vi "Stitch DAQ and Scope Data.vi"(8 "error in (no error)":errorcluster, 10 "Scope Ch1 (final A-B)":dbl[][](array[numeric]), 11 "DAQ DOD (final)":dbl[][](array[numeric])) -> (0 "error out":errorcluster, 3 "data & time array":dbl[][](array[numeric]))   [LabVIEW 2017, in "Processing.lvlib"]
doc: "Calculates the ambient voltage from 75% of the pretrigger data (pretrigger = 10% of \nthe full dataset), i.e. it's calculated from the first 7.5% of the data"
uses:
  Processing.lvlib
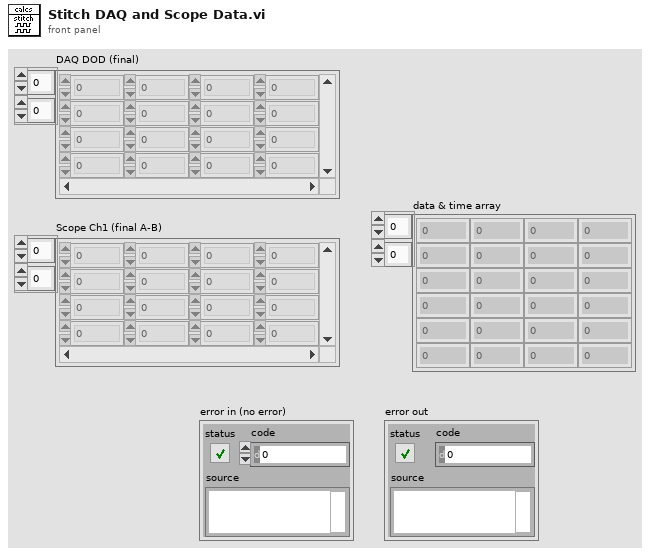
[diagram p1: front panel]
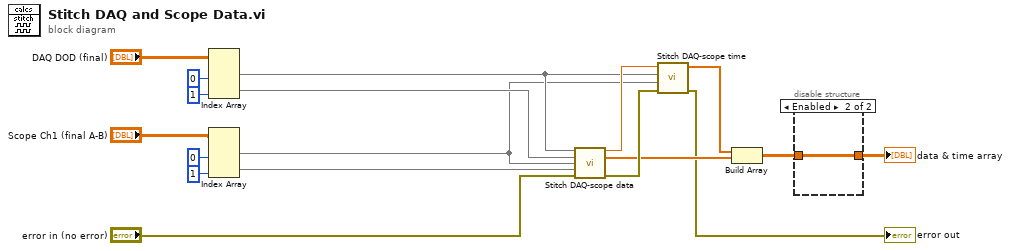
[diagram p0: block diagram]
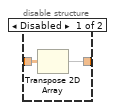
[diagram p2: hidden frame]
diagram:
  n1 = Index Array(array="DAQ DOD (final)", index (col) #1=0 ("disabled index (col)"), index (col) #2=1 ("index (col)")) -> (element #1=w11:dbl[], element #2=w10:dbl[])  [unwired: 2 in]
  n2 = Index Array(array="Scope Ch1 (final A-B)", index (col) #1=0 ("disabled index (col)"), index (col) #2=1 ("index (col)")) -> (element #1=w7:dbl[], element #2=w6:dbl[])  [unwired: 2 in]
  n3 = call "Stitch DAQ-scope data.vi"("DAQ time array (decimated)"=w11, "DAQ DOD (final)"=w10, "Scope Time arrays.Time axis"=w7, "Scope Data arrays.CH1 (final A-B)"=w6, "error in"="error in (no error)") -> (">> max scope time"=w15:dbl, "Stitched data array"=w16:dbl[], "error out"=w18:errorcluster)  [unwired: 8 in]
  n4 = call "Stitch DAQ-scope time.vi"("error in"=w18, "Scope Time arrays.Time axis"=w7, "DAQ time array (decimated)"=w11, "max scope time"=w15) -> ("error out"=→"error out":errorcluster, "Stiched scope-DAQ time array"=w14:dbl[])  [unwired: 6 in]
  n5 = Build Array(w14, w16) -> (w17:dbl[][])
  n6 = disable-structure shown="Enabled" {
    disable-tunnel: w17 -> [w20 w21]
    disable-tunnel: [w19 w21] -> w1
    frame Disabled {
      n7 = Transpose 2D Array(2D array=w20) -> (transposed array=w19:dbl[][])
    }
    frame Enabled {
    }
  }
  "data & time array" <- w1
